vi "Remove irrelevant data.vi"(9 "Input cluster":T1, 11 "XGrapher Range":T4) -> (1 "output cluster":T1, 3 "Output array size":i32)   [LabVIEW 2017]
uses:
  <vilib>/Utility/miscctls.llb/LVRangeTypeDef.ctl
  xcontrol/Interface VIs/Interface typedefs/Interface-Data format definition.ctl
  xcontrol/Typedefs/Xctl-XY data type definition.ctl
  xcontrol/Typedefs/Xctrl-ROI type enum.ctl
  <userlib>/_OpenG.lib/array/array.llb/Conditional Auto-Indexing Tunnel (SGL)__ogtk.vi
  xcontrol/XGrapher.xctl
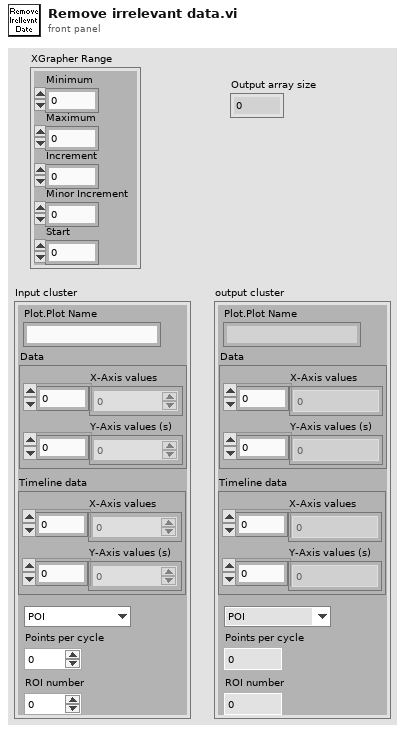
[diagram p1: front panel]
types:
  T1 = typedef "Interface-Data format definition.ctl" = cluster{"Plot.Plot Name":string, "Data":T2, "Timeline data":T2, "Type":T3, "Points per cycle":u16, "ROI number":u16}
  T2 = typedef "XGrapher.xctl/Xctl-XY data type definition.ctl" = cluster{"X-Axis values":sgl[], "Y-Axis values (s)":sgl[]}
  T3 = typedef "Xctrl-ROI type enum.ctl" = enum16{"POI", "Mini-scan", "Group"}
  T4 = typedef "LVRangeTypeDef.ctl" = cluster{"Minimum":dbl, "Maximum":dbl, "Increment":dbl, "Minor Increment":dbl, "Start":dbl}
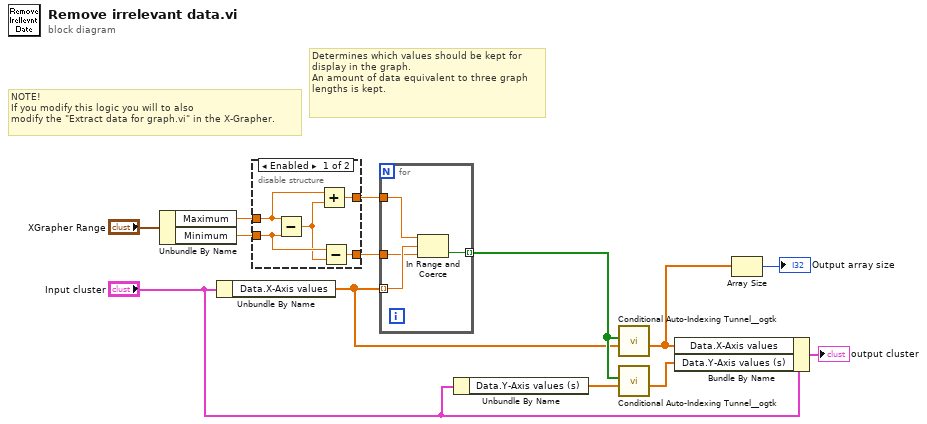
[diagram p0: block diagram]
diagram:
  # "NOTE!\nIf you modify this logic you will to also\nmodify the \"Extract data for graph.vi\" in the X-Grapher."
  # "Determines which values should be kept for display in the graph.\nAn amount of data equivalent to three graph lengths is kept."
  n1 = Unbundle By Name("XGrapher Range") -> ("Maximum"=w12:dbl, "Minimum"=w13:dbl)
  n2 = Unbundle By Name("Input cluster") -> ("Data.X-Axis values"=w3:sgl[])
  n3 = disable-structure shown="Enabled" {
    disable-tunnel: w12 -> [w18 w20]
    disable-tunnel: w13 -> [w17 w19]
    disable-tunnel: [w15 w20] -> w9
    disable-tunnel: [w14 w19] -> w10
    frame Enabled {
      n4 = Subtract(x=w18, y=w17) -> (x-y=w16:dbl)
      n5 = Add(x=w18, y=w16) -> (x+y=w15:dbl)
      n6 = Subtract(x=w17, y=w16) -> (x-y=w14:dbl)
    }
    frame Disabled {
    }
  }
  n7 = for {
    tunnel: w3 -> [w24] mode=indexing
    tunnel: [w23] -> w5 mode=indexing
    tunnel: w9 -> [w22]
    tunnel: w10 -> [w21]
    n8 = In Range and Coerce(upper limit=w22, x=w24, lower limit=w21) -> (In Range?=w23:bool)  [unwired: 1 out]
  }
  n9 = Unbundle By Name("Input cluster") -> ("Data.Y-Axis values (s)"=w8:sgl[])
  n10 = call-poly <userlib>:"Conditional Auto-Indexing Tunnel__ogtk.vi"("Array in"=w3, "Elements to keep"=w5) -> ("Filtered Array out"=w6:sgl[])  [unwired: 5 in]
  n11 = call-poly <userlib>:"Conditional Auto-Indexing Tunnel__ogtk.vi"("Array in"=w8, "Elements to keep"=w5) -> ("Filtered Array out"=w7:sgl[])  [unwired: 5 in]
  n12 = Bundle By Name(cluster="Input cluster", "Data.X-Axis values"=w6, "Data.Y-Axis values (s)"=w7) -> (→"output cluster":T1)
  n13 = Array Size(array=w6) -> (size(s)=→"Output array size":i32)
